vi "niScope Configure Trigger Immediate.vi"(0 "instrument handle":refnum<k15>, 11 "error in":errorcluster) -> (4 "instrument handle out":refnum<k15>, 15 "error out":errorcluster)   [LabVIEW 2011]
doc: "Configures common properties for immediate triggering. Immediate triggering means the digitizer triggers itself."
uses:
  niScope_32.dll
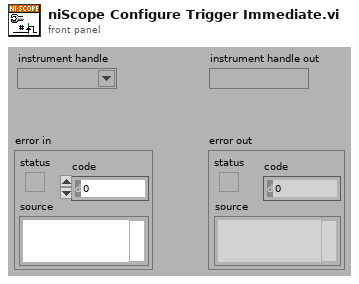
[diagram p1: front panel]
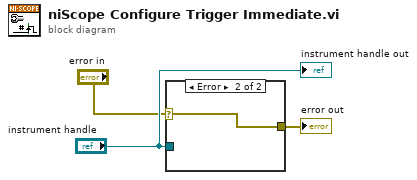
[diagram p0: block diagram]
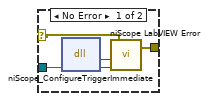
[diagram p2: hidden frame]
diagram:
  n1 = case shown="Error" "error in" {
    selector: "error in" -> [w4 w9]
    tunnel: [w5 w9] -> w2
    tunnel: "instrument handle" -> [w8 _]
    frame No Error {
      n2 = dll-call lib="niScope_*.*" fn="niScope_ConfigureTriggerImmediate"("instrument handle"=w8) -> ("status"=w7:i32, "instrument handle"=w6:u32)  [unwired: 3 in, 2 out]
      n3 = call "niScope LabVIEW Error.vi"("instrument handle"=w6, "niScope error code (0)"=w7, "error in (no error)"=w4) -> ("error out"=w5:errorcluster)  [unwired: 2 in]
    }
    frame Error {
    }
  }
  "error out" <- w2
  "instrument handle out" <- "instrument handle"
